vi "cw_4_3.vi"() -> ()   [LabVIEW 2022 SP3]
panel:
  out "lucky number":string
  in  "String":string="25.10.2001"
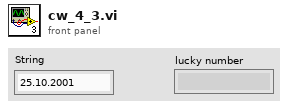
[diagram p1: front panel]
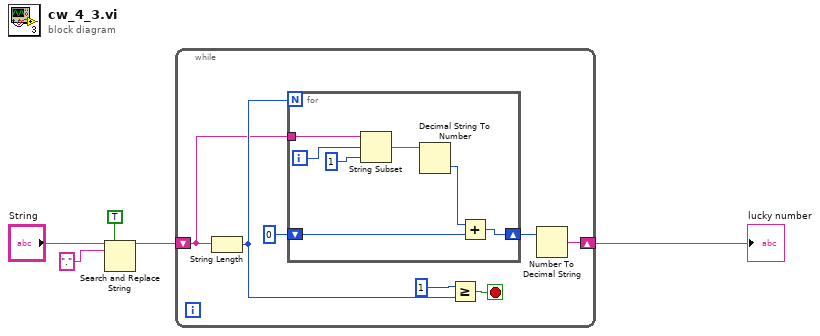
[diagram p0: block diagram]
diagram:
  n1 = Search and Replace String(replace all?=TRUE ("replace all? (F)"), input string="String", search string=".") -> (result string=w2:string)  [unwired: 5 in, 3 out]
  n2 = while {
    shift-right: [w8] -> w1
    shift-left: w2 -> [w9]
    stop <- w11 stop-if-true
    n3 = String Length(string=w9) -> (length=w10:i32)
    n4 = for {
      N: w10 -> [_]
      tunnel: w9 -> [w17]
      shift-right: [w15] -> w7
      shift-left: 0 -> [w13]
      i -> [w18]
      n5 = String Subset(string=w17, offset (0)=w18, length (rest)=1 ("length (rest)")) -> (substring=w16:string)
      n6 = Decimal String To Number(string=w16) -> (number=w14:i32)  [unwired: 2 in, 1 out]
      n7 = Add(x=w14, y=w13) -> (x+y=w15:i32)
    }
    n8 = Greater Or Equal?(x=1, y=w10) -> (x >= y?=w11:bool)
    n9 = Number To Decimal String(number=w7) -> (decimal integer string=w8:string)  [unwired: 1 in]
  }
  "lucky number" <- w1
